vi "Query Instrument Status.vi"(8 "error in (no error)":errorcluster, 10 "Instrument Status (0: Standard Event Status Enable Register)":u16(ring) items=["Standard Event Status Enable Register", "Service Request Enable Register", "Status Byte Register", "Standard Event Status Register", "Operation Complete"], 11 "VISA resource name":refnum<visa-resource-name>) -> (0 "error out":errorcluster, 2 "Register Value":u8, 3 "VISA resource name out":refnum<visa-resource-name>)   [LabVIEW 2017, in "HH PLI Series.lvlib"]
doc: "Queries different instrument status register.\n\n<b>Note</b>\nRefer to manual for details about the status register system."
uses:
  HH PLI Series.lvlib
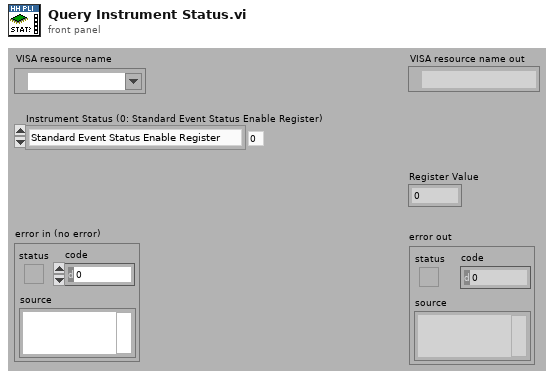
[diagram p1: front panel]
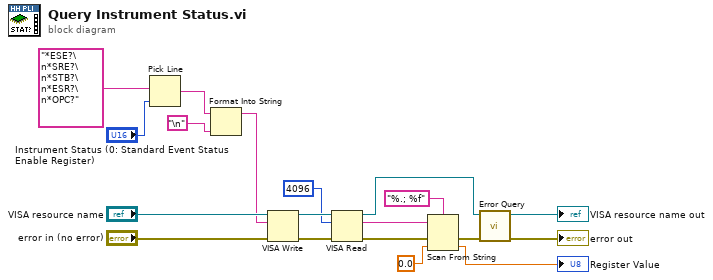
[diagram p0: block diagram]
diagram:
  n1 = Pick Line(multi-line string="*ESE?\n*SRE?\n*STB?\n*ESR?\n*OPC?", line index="Instrument Status (0: Standard Event Status Enable Register)") -> (output string=w2:string)  [unwired: 1 in]
  n2 = Format Into String(initial string=w2, "\n") -> (resulting string=w1:string)  [unwired: 2 in, 1 out]
  n3 = VISA Write(VISA resource name="VISA resource name", write buffer=w1, error in (no error)="error in (no error)") -> (VISA resource name out=w17:refnum<visa-resource-name>, error out=w16:errorcluster)  [unwired: 1 out]
  n4 = VISA Read(VISA resource name=w17, byte count=u32 4096, error in (no error)=w16) -> (VISA resource name out=w6:refnum<visa-resource-name>, read buffer=w14:string, error out=w12:errorcluster)  [unwired: 1 out]
  n5 = Scan From String(format string="%.; %f", input string=w14, error in=w12, default 1=0.0 ("default value 1")) -> (error out=w9:errorcluster, output 1=→"Register Value":dbl)  [unwired: 1 in, 2 out]
  n6 = call "Error Query.vi"("error in (no error)"=w9, "VISA resource name"=w6) -> ("error out"=→"error out":errorcluster, "VISA resource name out"=→"VISA resource name out":refnum<visa-resource-name>)  [unwired: 6 in, 2 out]
